vi "Baseline_subtraction.vi"() -> ()   [LabVIEW 2015]
uses:
  <vilib>/Analysis/baseanly.llb/Mean (DBL).vi
  <vilib>/Analysis/NI_AALBase.lvlib
panel:
  out "Baseline Subtracted":cluster{dbl[], dbl[]}[](graph)
  out "End part":cluster{dbl[], dbl[]}[](graph)
  in  "B0":dbl
  in  "B array":dbl[](array[numeric])
  in  "Averaged dt Out":dbl[][](array[numeric])
  in  "Averaged I(B) out":dbl[][](array[numeric])
  out "Total Average":T1(graph)
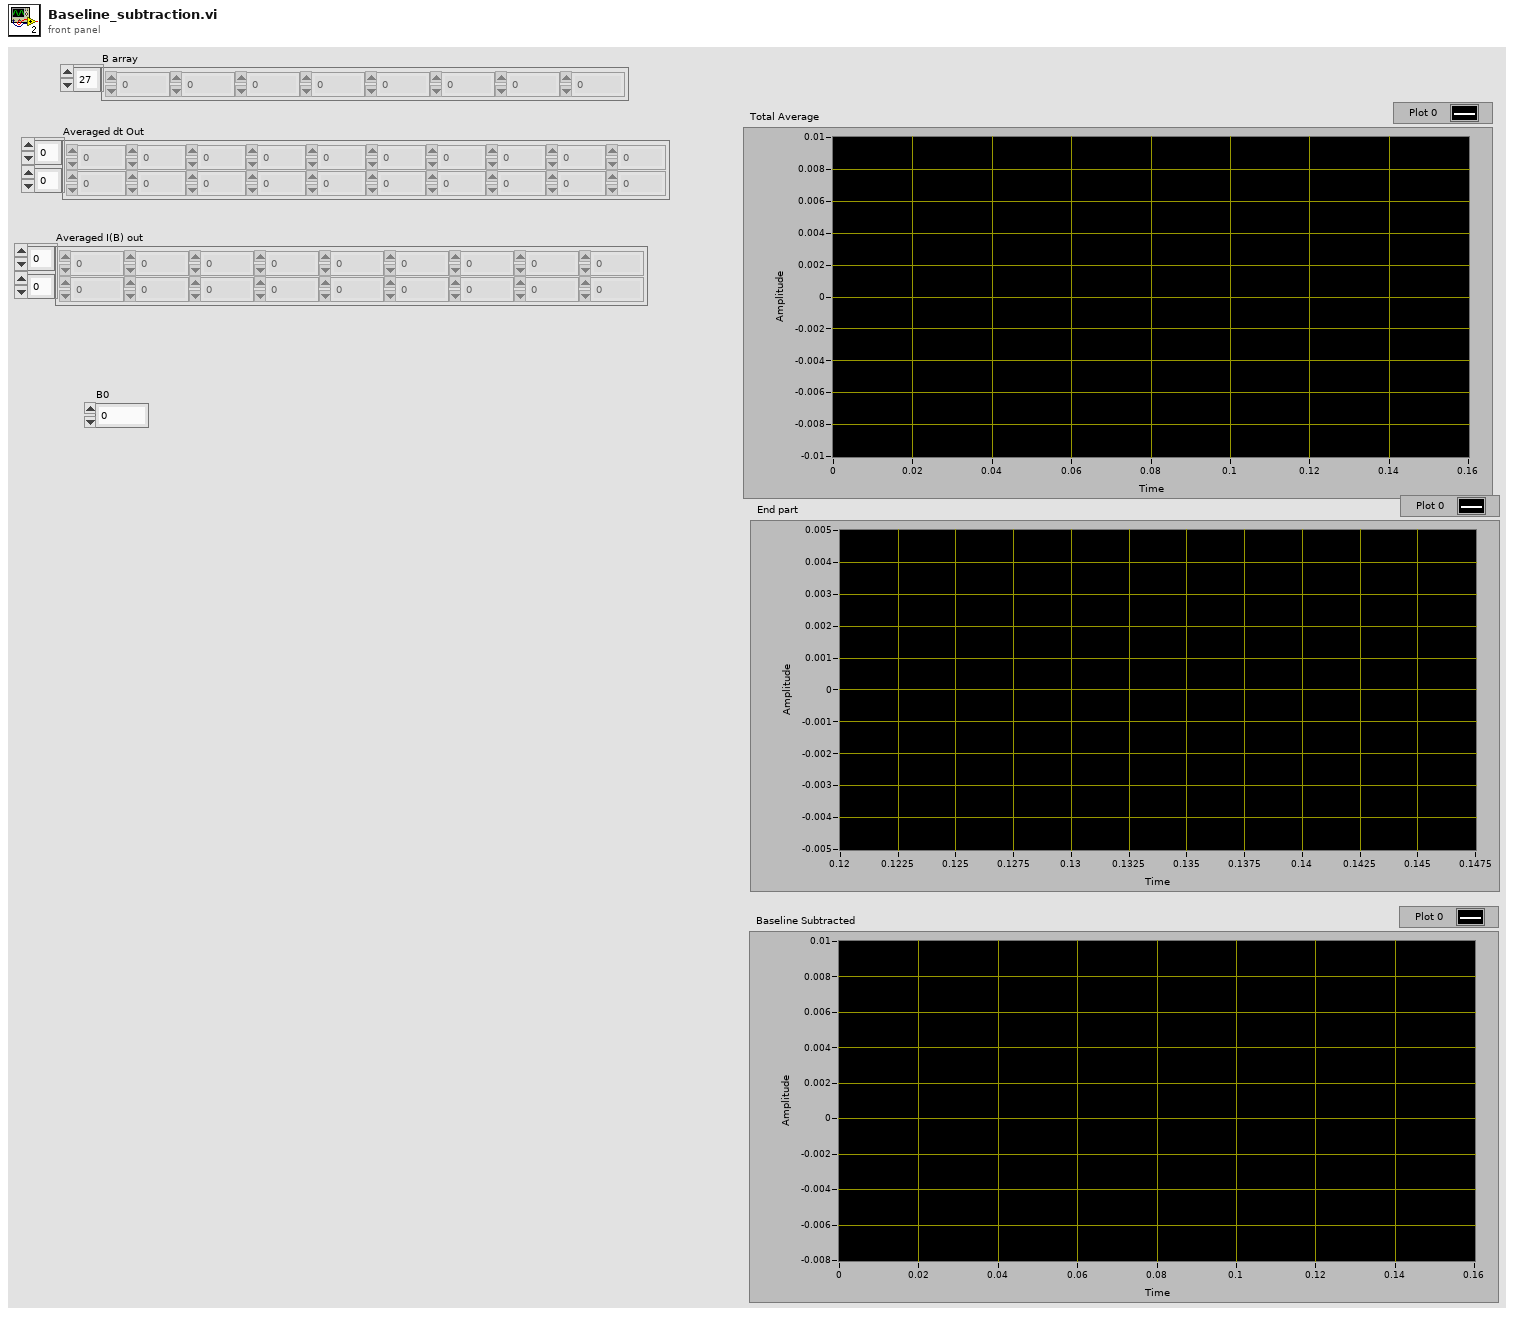
[diagram p1: front panel]
types:
  T1 = cluster{"Averaged dt in":dbl[], "Averaged I(B) In":dbl[]}[]
  T2 = cluster{"B array":dbl[], "Averaged I(B) out":dbl[]}
  T3 = cluster{"B array":dbl[], "Averaged I(B) out":dbl[]}[]
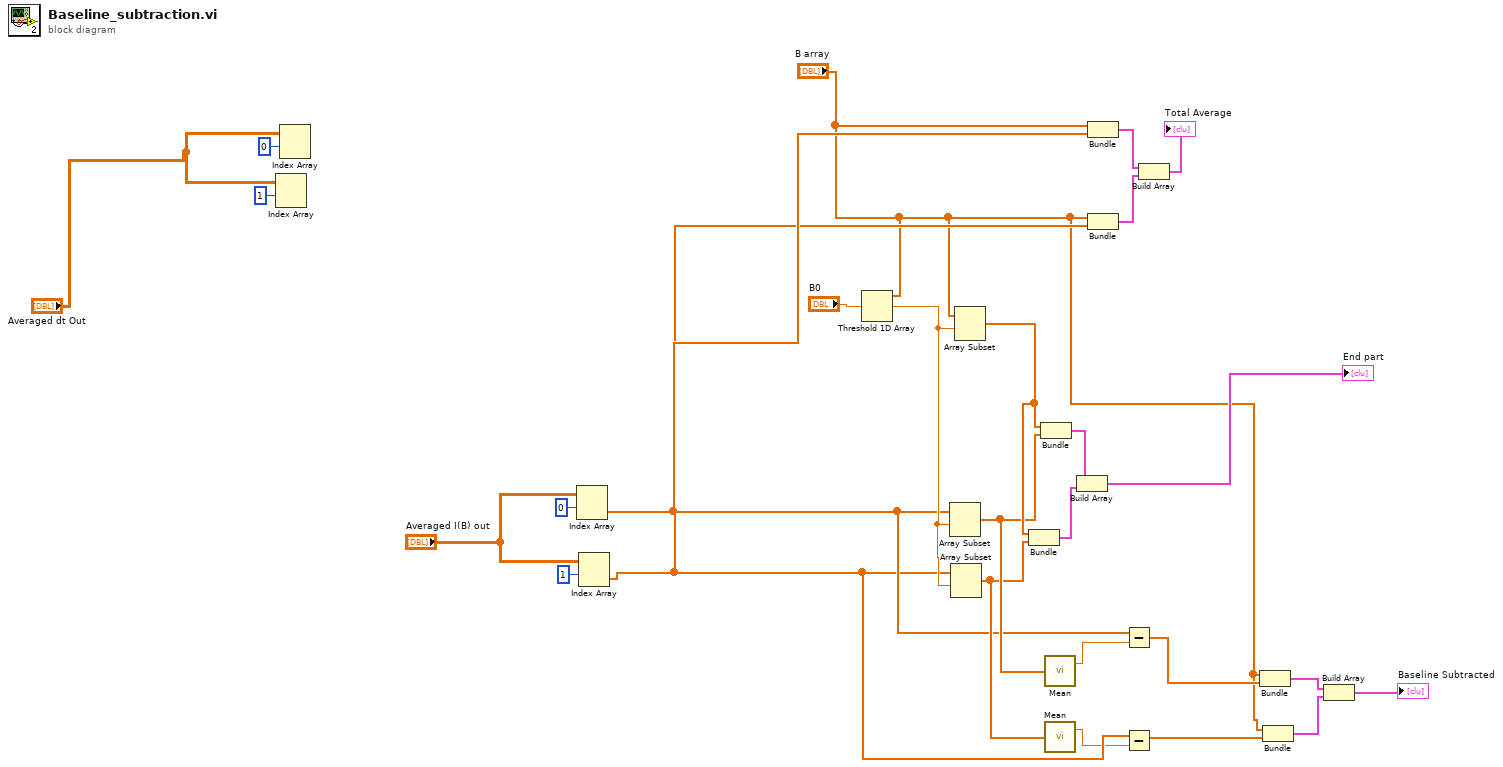
[diagram p0: block diagram]
diagram:
  n1 = Index Array(array="Averaged dt Out", index (row)=1) -> ()  [unwired: 1 in, 1 out]
  n2 = Index Array(array="Averaged dt Out", index (row)=0) -> ()  [unwired: 1 in, 1 out]
  n3 = Index Array(array="Averaged I(B) out", index (row)=0) -> (element=w10:dbl[])  [unwired: 1 in]
  n4 = Index Array(array="Averaged I(B) out", index (row)=1) -> (element=w8:dbl[])  [unwired: 1 in]
  n5 = Threshold 1D Array(2:"B0", 3:"B array") -> (0:w17:dbl)  [unwired: 1 in]
  n6 = Array Subset(array=w10, index=w17) -> (w12:dbl[])  [unwired: 1 in]
  n7 = Array Subset(array=w8, index=w17) -> (w11:dbl[])  [unwired: 1 in]
  n8 = Array Subset(array="B array", index=w17) -> (w16:dbl[])  [unwired: 1 in]
  n9 = Bundle(w16, w11) -> (w14:cluster{dbl[], dbl[]})  [unwired: 1 in]
  n10 = Bundle(w16, w12) -> (w15:cluster{dbl[], dbl[]})  [unwired: 1 in]
  n11 = call-poly <vilib>:"Mean.vi"("X"=w12) -> ("mean"=w9:dbl)  [unwired: 1 out]
  n12 = call-poly <vilib>:"Mean.vi"("X"=w11) -> ("mean"=w7:dbl)  [unwired: 1 out]
  n13 = Build Array(w15, w14) -> (→"End part":cluster{dbl[], dbl[]}[])
  n14 = Bundle("B array"="B array", "Averaged I(B) out"=w10) -> (w23:T2)  [unwired: 1 in]
  n15 = Bundle("B array"="B array", "Averaged I(B) out"=w8) -> (w22:T2)  [unwired: 1 in]
  n16 = Subtract(x=w10, y=w9) -> (x-y=w6:dbl[])
  n17 = Subtract(x=w8, y=w7) -> (x-y=w4:dbl[])
  n18 = Build Array(w23, w22) -> (→"Total Average":T3)
  n19 = Bundle("B array"="B array", w6) -> (w3:cluster{"B array":dbl[], dbl[]})  [unwired: 1 in]
  n20 = Bundle("B array"="B array", w4) -> (w2:cluster{"B array":dbl[], dbl[]})  [unwired: 1 in]
  n21 = Build Array(w3, w2) -> (→"Baseline Subtracted":cluster{"B array":dbl[], dbl[]}[])
